vi "Build Sim Device List_Orig.vi"() -> (3 "Sim Device List":T1)   [LabVIEW 2019]
uses:
  <vilib>/Utility/Data Type/NI_Data Type.lvlib
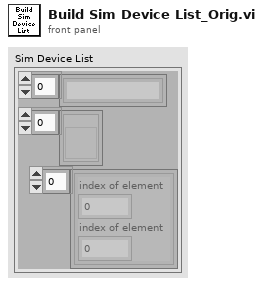
[diagram p1: front panel]
types:
  T1 = cluster{string[], refnum<vi>[], cluster{"index of element":i32, "index of element":i32}[]}
  T2 = cluster{"index of element":i32, "index of element":i32}
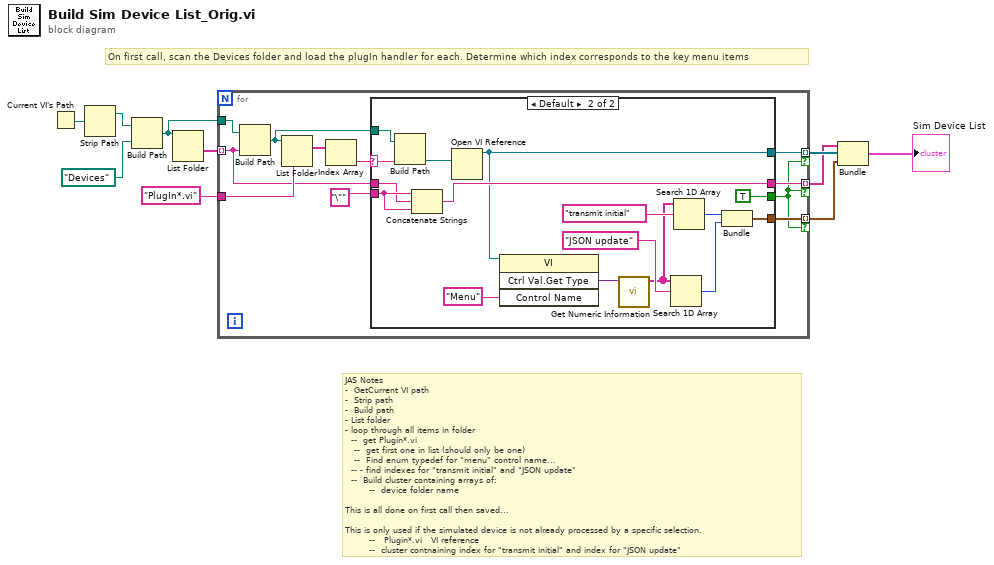
[diagram p0: block diagram]
diagram:
  # "JAS Notes\n-  GetCurrent VI path\n-  Strip path\n-  Build path\n- List folder\n- loop through all items in folder\n  --  get Plugin*.vi\n   --  get first one in list (should only be one)\n   --  Find enum typedef for \"menu\" control name... \n  -- - find indexes for \"transmit initial\" and \"JSON update\"\n  --  Build cluster containing arrays of:\n        --  device folder name\n\nThis is all done on first call then saved...\n\nThis is only used if the simulated device is not already processed by a specific selection.\n        --   Plugin*.vi   VI reference\n        --  cluster contnaining index for \"transmit initial\" and index for \"JSON update\""
  # "On first call, scan the Devices folder and load the plugIn handler for each. Determine which index corresponds to the key menu items"
  n1 = Current VI's Path() -> (path=w1:path)
  n2 = Strip Path(path=w1) -> (stripped path=w2:path)  [unwired: 1 out]
  n3 = Build Path(base path=w2, name or relative path=path "Devices") -> (appended path=w4:path)
  n4 = List Folder(path=w4) -> (folder names=w3:string[])  [unwired: 3 in, 3 out]
  n5 = for {
    tunnel: w3 -> [w17] mode=indexing
    tunnel: w4 -> [w21]
    tunnel: "PlugIn*.vi" ("pattern") -> [w20]
    tunnel: [w16] -> w7 mode=indexing if=w11
    tunnel: [w15] -> w6 mode=indexing if=w11
    tunnel: [w12] -> w9 mode=indexing if=w11
    n6 = Build Path(base path=w21, name or relative path=w17) -> (appended path=w14:path)
    n7 = List Folder(path=w14, pattern=w20) -> (filenames=w19:string[])  [unwired: 2 in, 3 out]
    n8 = Index Array(array=w19) -> (element=w18:string)  [unwired: 1 in]
    n9 = case shown="Default" w18 {
      selector: w18 -> [_ w36]
      tunnel: [_ w29] -> w16
      tunnel: w17 -> [_ w31]
      tunnel: [_ w32] -> w15
      tunnel: [_ TRUE] -> w11
      tunnel: w14 -> [_ w35]
      tunnel: "\"" -> [_ w33]
      tunnel: [_ w22] -> w12
      frame "", "Tmpl_PanelSim_Global.vi" {
        # "not found\nor tmpl"
      }
      frame Default {
        n10 = Build Path(base path=w35, name or relative path=w36) -> (appended path=w34:path)
        n11 = Concatenate Strings(w33, w31, w33) -> (w32:string)
        n12 = Open VI Reference(vi path=w34) -> (vi reference=w29:refnum<vi>)  [unwired: 5 in, 1 out]
        n13 = invoke class="VI" method="Ctrl Val.Get Type"(reference=w29, "Control Name"="Menu" ("whole match")) -> ("Ctrl Val.Get Type"=w30:variant)  [unwired: 2 in, 3 out]
        n14 = call <vilib>:"Get Numeric Information.vi"("variant"=w30) -> ("enum names"=w25:string[])  [unwired: 7 in, 3 out]
        n15 = Search 1D Array(1D array=w25, element="JSON update" ("whole match")) -> (index of element=w23:i32)  [unwired: 1 in]
        n16 = Search 1D Array(1D array=w25, element="transmit initial" ("whole match")) -> (index of element=w24:i32)  [unwired: 1 in]
        n17 = Bundle("index of element"=w24, "index of element"=w23) -> (w22:T2)  [unwired: 1 in]
      }
    }
  }
  n18 = Bundle(w6, w7, w9) -> (→"Sim Device List":T1)  [unwired: 1 in]
